vi "Configure Measurement.vi"(0 "reference in":refnum<class "BKP-891 LCR Meter.lvclass">, 2 "LR Mode":T1, 5 "error in (no error)":errorcluster) -> (14 "reference out":refnum<class "BKP-891 LCR Meter.lvclass">, 19 "error out":errorcluster)   [LabVIEW 2018, in "BKP-891 LCR Meter.lvclass"]
uses:
  BKP-891 LCR Meter.lvclass
  controls/LR Mode.ctl
  <instrlib>/BK Precision 891/BK Precision 891.lvlib
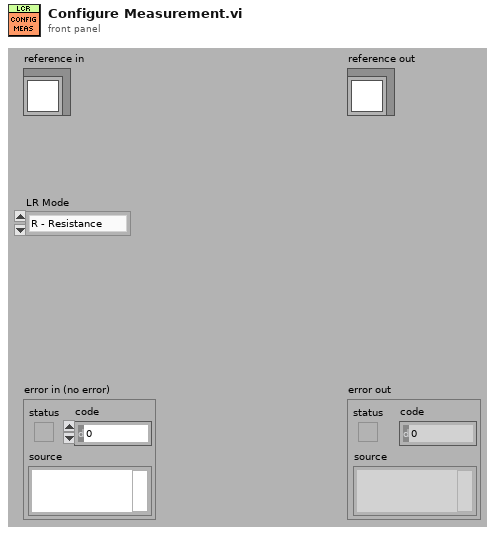
[diagram p1: front panel]
types:
  T1 = typedef "LR Mode.ctl" = enum16{"R - Resistance", "L - Inductance"}
  T2 = typedef "BKP-891 LCR Meter.lvclass/ObjectAttributes.ctl" = cluster{"VISA resource name":refnum<visa-resource-name>, "Simulated?":bool, "Latest Values":dbl[], "Signal List":T3[], "Tare Offset":dbl[], "Range":u16, "Measurement Speed":u16, "Function":u16, "Signal Frequency (Hz)":dbl, "Signal Level (Vrms)":u8, "UVW Mode":enum16{"UV", "UW", "VW", "None"}, "LR Mode":T1, "Primary Parameter":string, "Secondary Parameter":string}
  T3 = typedef "IO Signal List.ctl" = enum16{"Timestamp", "PSU_FB_U_VDC", "PSU_FB_I_AMP", "PSU_FB_W_WATT", "PSU_CMD_U_VDC", "PSU_CMD_I_AMP", "PSU_CMD_OUTPUT", "LCR_PRIMARY", "LCR_SECONDARY", "UV_R_Ohm", "UW_R_Ohm", "VW_R_Ohm", "UV_L_H", "UW_L_H", "VW_L_H", "U_U_VDC", "V_U_VDC", "W_U_VDC", "U_I_AMP", "V_I_AMP", "W_I_AMP", "PWM_CMD_DC_%", "PWM_CMD_VDC", "PWM_CMD_Hz", "PWM_FB_DC_%", "PWM_FB_VDC", "PWM_FB_Hz", "DO_RELAY_U_LCR_A", "DO_RELAY_V_LCR_A", "DO_RELAY_V_LCR_B", "DO_RELAY_W_LCR_B", "DIFF_UV_UW_L_H", "DIFF_UV_VW_L_H", "DIFF_UW_VW_L_H", "DIFF_UV_UW_R_Ohm", "DIFF_UV_VW_R_Ohm", "DIFF_UW_VW_R_Ohm", "DIFF_UV_U_VDC", "DIFF_UW_U_VDC", "DIFF_VW_U_VDC"}
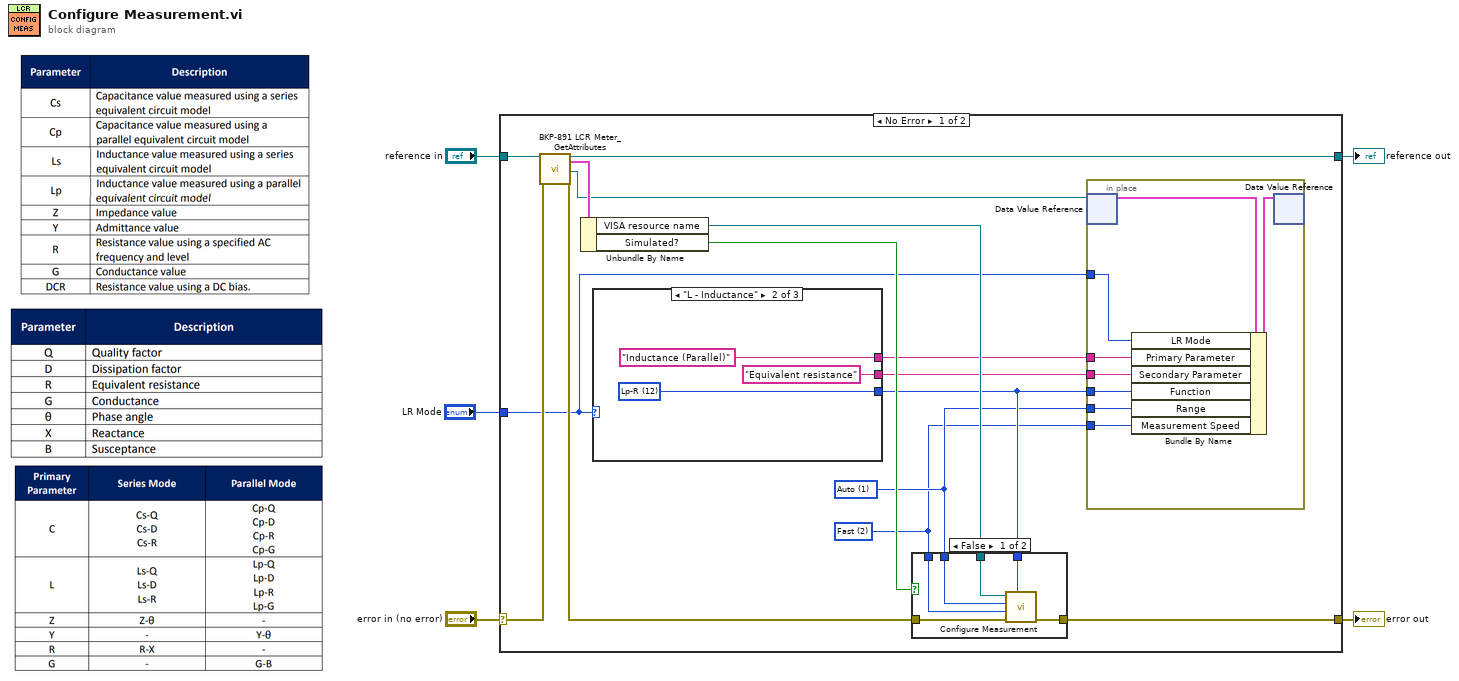
[diagram p0: block diagram]
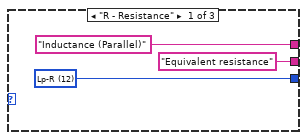
[diagram p2: hidden frame]
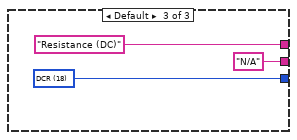
[diagram p3: hidden frame]
diagram:
  n1 = case shown="No Error" "error in (no error)" {
    selector: "error in (no error)" -> [w20 w46]
    tunnel: [w14 w46] -> w4
    tunnel: [w17 w45] -> w2
    tunnel: "reference in" -> [w18 w45]
    tunnel: "LR Mode" -> [w6 _]
    frame No Error {
      w10 = u16 1 items=["Hold", "Auto"] ("Range (1:Auto)")
      w9 = u16 2 items=["Slow"=1, "Fast"=2] ("Measurement Speed (2:Fast)")
      n2 = call "BKP-891 LCR Meter_GetAttributes.vi"("reference in"=w18, "error in (no error)"=w20) -> ("reference out"=w17:refnum<class "BKP-891 LCR Meter.lvclass">, "Data"=w19:T2, "DataRef"=w13:refnum<data-value>, "error out"=w15:errorcluster)  [unwired: 14 in]
      n3 = Unbundle By Name(w19) -> ("VISA resource name"=w16:refnum<visa-resource-name>, "Simulated?"=w12:bool)
      n4 = case shown="\"L - Inductance\"" w6 {
        tunnel: [w23 w26 w29] -> w11
        tunnel: ["Inductance (Parallel)" "Inductance (Parallel)" "Resistance (DC)"] -> w8
        tunnel: ["Equivalent resistance" "Equivalent resistance" "N/A"] -> w7
        frame "R - Resistance" {
          w23 = u16 12 items=["Cs-Q", "Cs-D", "Cs-R", "Cp-Q", "Cp-D", "Cp-R", "Cp-G", "Ls-Q", "Ls-D", "Ls-R", "Lp-Q", "Lp-D", "Lp-R", "Lp-G", "Z-th", "Y-th", "R-X", "G-B", "DCR"] ("Function (4: Cp-D)")
        }
        frame "L - Inductance" {
          w26 = u16 12 items=["Cs-Q", "Cs-D", "Cs-R", "Cp-Q", "Cp-D", "Cp-R", "Cp-G", "Ls-Q", "Ls-D", "Ls-R", "Lp-Q", "Lp-D", "Lp-R", "Lp-G", "Z-th", "Y-th", "R-X", "G-B", "DCR"] ("Function (4: Cp-D)")
        }
        frame Default {
          w29 = u16 18 items=["Cs-Q", "Cs-D", "Cs-R", "Cp-Q", "Cp-D", "Cp-R", "Cp-G", "Ls-Q", "Ls-D", "Ls-R", "Lp-Q", "Lp-D", "Lp-R", "Lp-G", "Z-th", "Y-th", "R-X", "G-B", "DCR"] ("Function (4: Cp-D)")
        }
      }
      n5 = case shown="False" w12 {
        tunnel: w16 -> [w35 _]
        tunnel: w15 -> [w34 w36]
        tunnel: [w33 w36] -> w14
        tunnel: w11 -> [w32 _]
        tunnel: w10 -> [w31 _]
        tunnel: w9 -> [w30 _]
        frame False {
          n6 = call <instrlib>:"Configure Measurement.vi"("Function (4: Cp-D)"=w32, "error in (no error)"=w34, "Measurement Speed (2:Fast)"=w30, "Range (1:Auto)"=w31, "VISA resource name"=w35) -> ("error out"=w33:errorcluster)  [unwired: 5 in, 1 out]
        }
        frame True {
        }
      }
      n7 = in-place {
        in-place-border: w11 -> [w42]
        in-place-border: w10 -> [w41]
        in-place-border: w9 -> [w40]
        in-place-border: w8 -> [w39]
        in-place-border: w7 -> [w38]
        in-place-border: w6 -> [w37]
        n8 = in-place-dvr #1(w13) -> (w44:T2)  [unwired: 1 out]
        n9 = Bundle By Name(cluster=w44, "LR Mode"=w37, "Primary Parameter"=w39, "Secondary Parameter"=w38, "Function"=w42, "Range"=w41, "Measurement Speed"=w40) -> (w43:T2)
        n10 = in-place-dvr #1(w43) -> ()  [unwired: 2 out]
      }
    }
    frame Error {
    }
  }
  "error out" <- w4
  "reference out" <- w2
